vi "Set 16 symbols.vi"(8 "error in (no error)":errorcluster, 10 "16 symbols":bool=TRUE, 11 "niDTS WLAN Dut in":refnum<class "niDTS WLAN Dut.lvclass">) -> (0 "error out":errorcluster, 3 "niDTS WLAN Dut out":refnum<class "niDTS WLAN Dut.lvclass">)   [LabVIEW 2015, in "niDTS WLAN.lvlib" / "niDTS WLAN Dut.lvclass"]
doc: "Specifies if 16 symbols of payload length should be used. If set to TRUE, this sets the payload length, in bytes, to 16 symbols according to the standard, rate, bandwidth and streams. If Payload Length limit has been set, the caluclated payload length is capped at the Payload Length Limit."
uses:
  niDTS WLAN Dut.lvclass
  niDTS WLAN Dut.lvclass/niDTS WLAN Dut.ctl
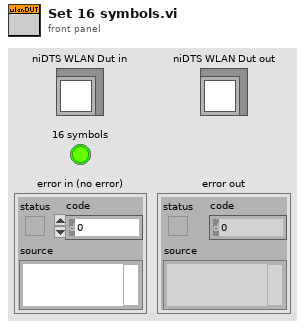
[diagram p1: front panel]
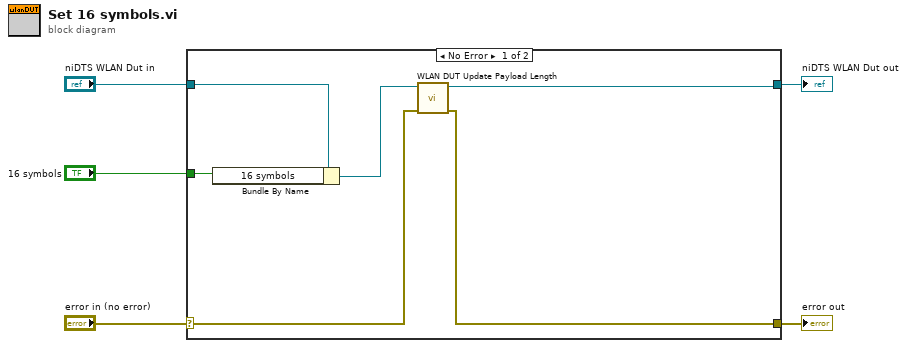
[diagram p0: block diagram]
diagram:
  n1 = case shown="No Error" "error in (no error)" {
    selector: "error in (no error)" -> [w8 w12]
    tunnel: [w7 w12] -> w4
    tunnel: [w6 w13] -> w2
    tunnel: "niDTS WLAN Dut in" -> [w10 w13]
    tunnel: "16 symbols" -> [w11 _]
    frame No Error {
      n2 = Bundle By Name(cluster=w10, "16 symbols"=w11) -> (w9:refnum<class "niDTS WLAN Dut.lvclass">)
      n3 = call-dynamic "WLAN DUT Update Payload Length.vi"("error in (no error)"=w8, "niDTS WLAN DUT in"=w9) -> ("error out"=w7:errorcluster, "niDTS WLAN DUT out"=w6:refnum<class "niDTS WLAN Dut.lvclass">)  [unwired: 8 in]
    }
    frame Error {
    }
  }
  "error out" <- w4
  "niDTS WLAN Dut out" <- w2
